vi "MoveandWait.vi"(3 "Motion Settings":T1={"No Motion?"=FALSE, "Motion System"=enum."No Motion Card", "Motion Bd ID"=1, "Motion Profile"="SMAC1", "# Axis"=1, "Reverse Z axis?"=TRUE, "SMAC Axis"=0, "scan pair"=enum."y-(x) scan", "RT fps"=6.0, "Steps per mm"=[1000, 1000, 1000, 1000], "Motor Parameters"={"velocity ct/s"=[10000.0, 10000.0, 10000.0, 50000.0], "accel ct/s^2"=[50000.0, 50000.0, 50000.0, 200000.0]}, "One Way Scan"=FALSE, "Reverse One Way Scan"=FALSE, "Global Position (mm)"=[], "Plane"=0, "Distance between\nscan lines (um)"=0.0, "Distance between\nscan planes (um)"=0.0, "number of scan planes"=1, "Total steps in line"=0, "Xtra plane\ndistance  (um)"=100, "Xtra planes "=1, "Add Axis"=FALSE, "overshoot cts"=200, "BKPT Shift"=0, "Scan Start Time (ms)"=0, "ESP VISA"="GPIB::1::INSTR", "3rd Axis"=1, "GL Ref Out"=refnum, "Galil Address"=""} {"3rd Axis" items=["x", "y", "z", "w"]; "Xtra planes" min=1; "Xtra plane\ndistance  (um)" min=0; "Distance between\nscan planes (um)" format="%.2f"; "Distance between\nscan lines (um)" format="%.2f"; "SMAC Axis" items=["None"=0, "Axis 1"=1, "Axis 2"=2, "Axis 3"=3, "Axis 4"=4, "Axis 5"=5, "Axis 6"=6, "Axis 7"=7, "Axis 8"=8, "Vector Space 1"=17, "Vector Space 2"=18, "Vector Space 3"=19, "Vector Space 4"=20]; "Motion Bd ID" min=1 max=32 step=1}, 4 "time to wait (ms)":dbl format="%.2f", 5 "steps to move":dbl format="%.2f", 6 "Axis":i32, 7 "Move and Wait?":bool) -> ()   [LabVIEW 2022 SP3]
uses:
  ScanningControl/Motion Controllers/NI_controller/-NI_MotionRoutines/MotionParameters.ctl
  ScanningControl/Motion Controllers/NI_controller/-NI_MotionRoutines/MotionSys.ctl
  ScanningControl/Motion Controllers/-MotionRoutines/ScanAxis.ctl
  ScanningControl/Motion Controllers/-MotionRoutines/3rdAxis.ctl
panel:
  # "1-D and 2-D B scan settings"
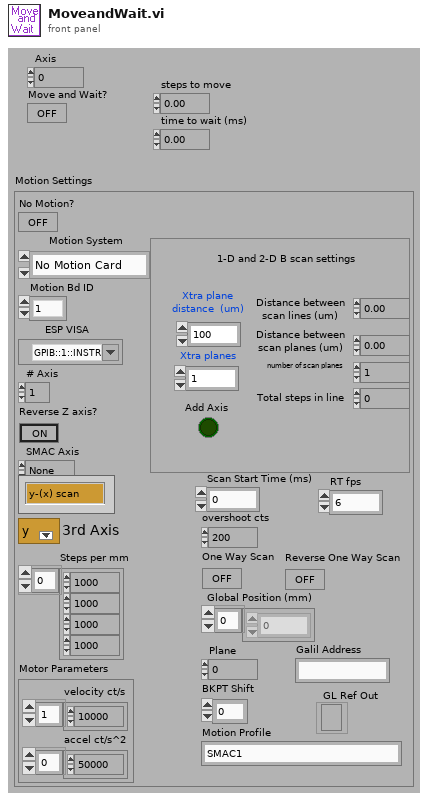
[diagram p1: front panel]
types:
  T1 = typedef "MotionParameters.ctl" = cluster{"No Motion?":bool, "Motion System":T2, "Motion Bd ID":u8, "Motion Profile":string, "# Axis":i8, "Reverse Z axis?":bool, "SMAC Axis":u16, "scan pair":T3, "RT fps":sgl, "Steps per mm":i32[], "Motor Parameters":cluster{"velocity ct/s":dbl[], "accel ct/s^2":dbl[]}, "One Way Scan":bool, "Reverse One Way Scan":bool, "Global Position (mm)":dbl[], "Plane":i32, "Distance between\nscan lines (um)":sgl, "Distance between\nscan planes (um)":sgl, "number of scan planes":i32, "Total steps in line":i32, "Xtra plane\ndistance  (um)":i32, "Xtra planes ":i32, "Add Axis":bool, "overshoot cts":i32, "BKPT Shift":i32, "Scan Start Time (ms)":u32, "ESP VISA":refnum<visa-resource-name>, "3rd Axis":T4, "GL Ref Out":refnum<k7>, "Galil Address":string}
  T2 = typedef "MotionSys.ctl" = enum16{"MM3000", "NI 735x", "Newport ESP", "No Motion Card", "Galil"}
  T3 = typedef "ScanAxis.ctl" = enum16{"y-(x) scan", "x-(y) scan", "z-(x) scan", "z-(y) scan", "y-(z) scan", "x-(z) scan", "w-(x) scan", "w-(y) scan", "w-(z) scan", "x-(w) scan", "y-(w) scan", "z-(w) scan"}
  T4 = typedef "3rdAxis.ctl" = u16
  T5 = enum16{"Absolute Position", "Relative Position", "Velocity", "Relative to Cap Pos", "Modulus Position", "Absolute Contouring", "Relative Contouring"}
  T6 = typedef "GL Axis Control.ctl" = u16
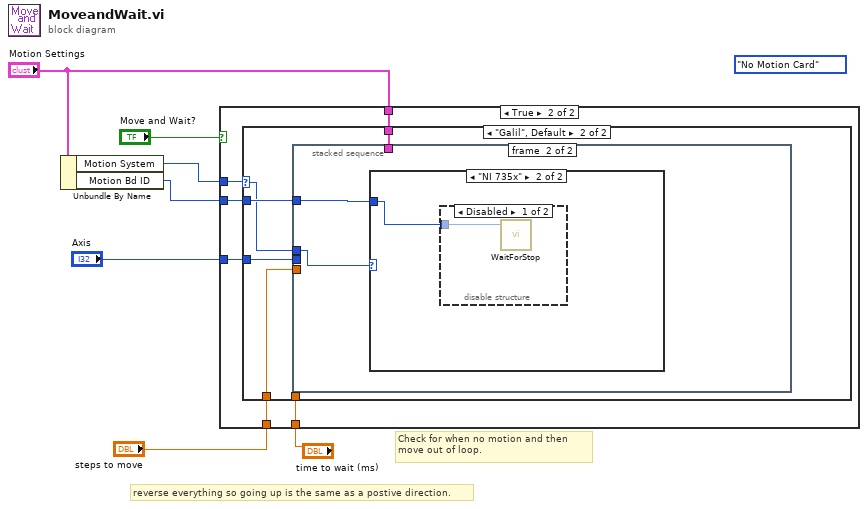
[diagram p0: block diagram]
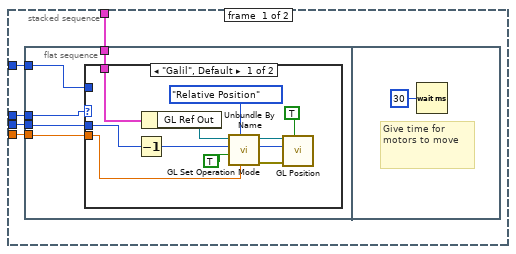
[diagram p4: hidden frame]
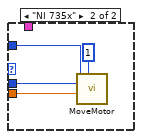
[diagram p5: hidden frame]
diagram:
  (unwired) MotionSys."No Motion Card" ("Motion System")
  # "Check for when no motion and then \nmove out of loop."
  # "reverse everything so going up is the same as a postive direction."
  n1 = Unbundle By Name("Motion Settings") -> ("Motion System"=w2:T2, "Motion Bd ID"=w1:u8)
  n2 = case shown="True" "Move and Wait?" {
    tunnel: "time to wait (ms)" -> [_ w13]
    tunnel: "steps to move" -> [_ w12]
    tunnel: "Axis" -> [_ w11]
    tunnel: w2 -> [_ w10]
    tunnel: w1 -> [_ w9]
    tunnel: "Motion Settings" -> [_ w8]
    frame False {
    }
    frame True {
      n3 = case shown="\"Galil\", Default" w10 {
        selector: w10 -> [_ w14]
        tunnel: w13 -> [_ _]
        tunnel: w12 -> [_ w17]
        tunnel: w11 -> [_ w18]
        tunnel: w9 -> [_ w16]
        tunnel: w8 -> [_ w15]
        frame "No Motion Card" {
        }
        frame "Galil", Default {
          n4 = stacked-sequence {
            tunnel: w18 -> [w22 _]
            tunnel: w17 -> [w23 _]
            tunnel: w16 -> [w21 w46]
            tunnel: w14 -> [w20 w45]
            tunnel: w15 -> [w19 _]
            frame #0 {
              n5 = flat-sequence {
                tunnel: w23 -> [w28]
                tunnel: w22 -> [w27]
                tunnel: w21 -> [w26]
                tunnel: w20 -> [w25]
                tunnel: w19 -> [w24]
                frame #0 {
                  n6 = case shown="\"Galil\", Default" w25 {
                    tunnel: w28 -> [w37 w42]
                    tunnel: w27 -> [w36 w41]
                    tunnel: w26 -> [_ w40]
                    tunnel: w24 -> [w35 _]
                    frame "Galil", Default {
                      n7 = Decrement(x=w36) -> (x-1=w30:i32)
                      n8 = Unbundle By Name(w35) -> ("GL Ref Out"=w39:refnum<k7>)
                      n9 = call "GL Set Operation Mode.vi"("position cts (abs/rel)"=w37, "Position Mode (Absolute)"=T5."Relative Position", "Start Now?"=TRUE, "Axis"=w30, "Galil.IGalil"=w39) -> ("error out"=w32:errorcluster, "Axis Out Output"=w29:T6, "Galil Out"=w33:refnum<k7>)  [unwired: 4 in]
                      n10 = call "GL Position.vi"("Wait for Motion Complete"=TRUE, "error in (no error)"=w32, "Axis"=w29, "Galil.IGalil"=w33) -> ()  [unwired: 2 in, 4 out]
                    }
                    frame "NI 735x" {
                      n11 = call "MoveMotor.vi"("Position Mode (Absolute)"=1, "Target Position (0)"=w42, "Axis or Vector Space"=w41, "Motion Bd ID"=w40) -> ()  [unwired: 1 in, 7 out]
                    }
                  }
                }
                frame #1 {
                  # "Give time for motors to move"
                  n12 = Wait (ms)(milliseconds to wait=30) -> ()  [unwired: 1 out]
                }
              }
            }
            frame #1 {
              n13 = case shown="\"NI 735x\"" w45 {
                tunnel: w46 -> [_ w47]
                frame "Galil", Default {
                }
                frame "NI 735x" {
                  n14 = disable-structure shown="Disabled" {
                    disable-tunnel: w47 -> [w48 _]
                    frame Disabled {
                      n15 = call "WaitForStop.vi"("Board ID"=w48) -> ()  [unwired: 2 in, 3 out]
                    }
                    frame Enabled {
                    }
                  }
                }
              }
            }
          }
        }
      }
    }
  }
